vi "ReadWriteClassAttributeOld.vi"(5 "error in (no error)":errorcluster) -> (19 "error out":errorcluster)   [LabVIEW 2020, in "G#MethodTemplates.lvclass"]
uses:
  G#MethodTemplates.lvclass
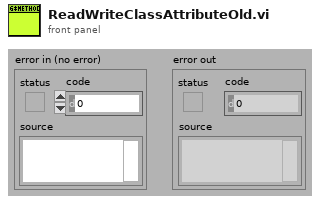
[diagram p1: front panel]
types:
  T1 = typedef "G#MethodTemplates.lvclass/ClassAttributes.ctl" = cluster{"Dummy":bool}
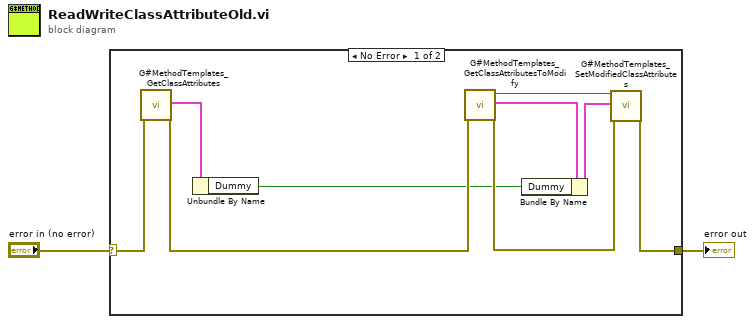
[diagram p0: block diagram]
diagram:
  n1 = case shown="No Error" "error in (no error)" {
    selector: "error in (no error)" -> [w6 w12]
    tunnel: [w8 w12] -> w1
    frame No Error {
      n2 = call "G#MethodTemplates_GetClassAttributes.vi"("error in (no error)"=w6) -> ("class attributes"=w3:T1, "error out"=w5:errorcluster)  [unwired: 15 in, 2 out]
      n3 = Unbundle By Name(w3) -> ("Dummy"=w4:bool)
      n4 = call "G#MethodTemplates_GetClassAttributesToModify.vi"("error in (no error)"=w5) -> ("reference out"=w9:refnum<class "G#BaseTemplateG3.lvclass">, "class attributes"=w11:T1, "error out"=w7:errorcluster)  [unwired: 13 in, 3 out]
      n5 = Bundle By Name(cluster=w11, "Dummy"=w4) -> (w10:T1)
      n6 = call "G#MethodTemplates_SetModifiedClassAttributes.vi"("reference in"=w9, "attributes"=w10, "error in (no error)"=w7) -> ("error out"=w8:errorcluster)  [unwired: 15 in, 1 out]
    }
    frame Error {
    }
  }
  "error out" <- w1
